vi "Add record to CSV.vi"(8 "error in":errorcluster, 10 "New row":string[](array[string]), 11 "CSV file":path) -> (0 "error out":errorcluster)   [LabVIEW 2013]
uses:
  <vilib>/Utility/file.llb/Read From Spreadsheet File (string).vi
  <vilib>/Utility/file.llb/Write To Spreadsheet File (string).vi
panel:
  out "Lines and rows":i32[](array[numeric])=[1917, 7]
  out "Spread Sheet Display":string[][](array[string])
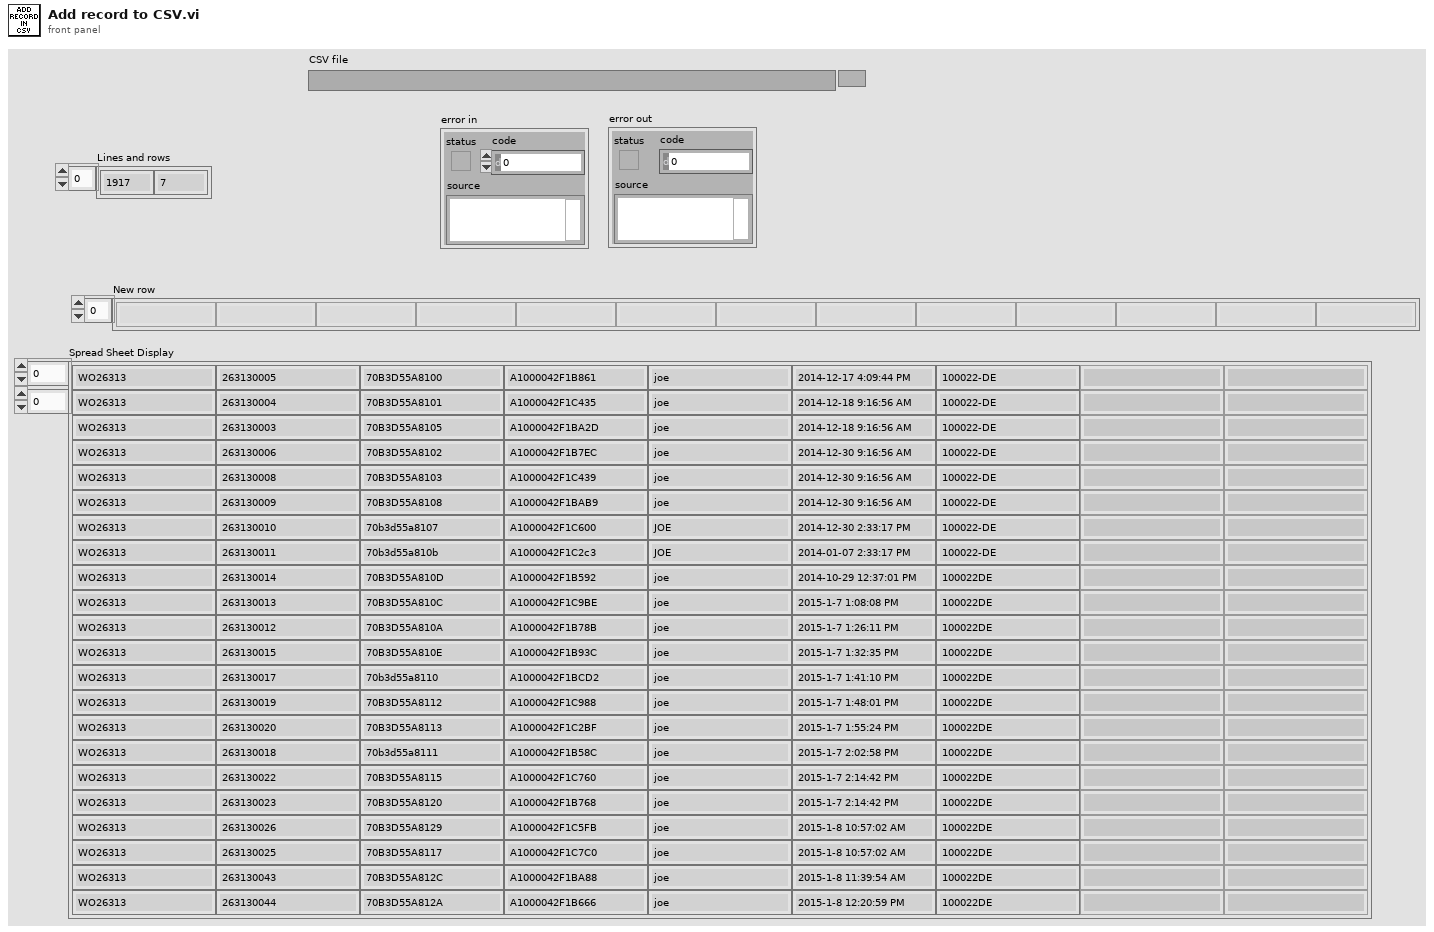
[diagram p1: front panel]
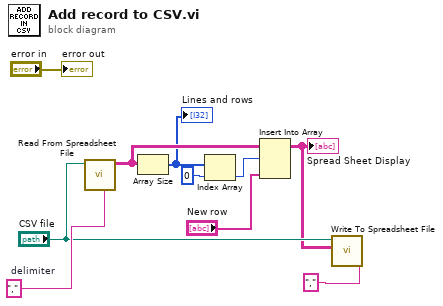
[diagram p0: block diagram]
diagram:
  w10 = ","  # delimiter
  n1 = call-poly <vilib>:"Read From Spreadsheet File.vi"("delimiter (\\t)"=w10, "file path (dialog if empty)"="CSV file") -> ("all rows"=w8:string[][])  [unwired: 5 in, 4 out]
  n2 = Array Size(array=w8) -> (size(s)=w7:i32[])
  "Lines and rows" <- w7
  n3 = Index Array(array=w7, index=0) -> (element=w5:i32)
  n4 = Insert Into Array(array=w8, index (row)=w5, new element="New row") -> (w2:string[][])  [unwired: 1 in]
  "Spread Sheet Display" <- w2
  n5 = call-poly <vilib>:"Write To Spreadsheet File.vi"("delimiter (\\t)"="," ("delimiter (\\t)"), "2D data"=w2, "file path (dialog if empty)"="CSV file") -> ()  [unwired: 5 in, 1 out]
  "error out" <- "error in"
